vi "Configure_Self_Test.vi"(7 "I2C Channel":u8, 8 "error in":errorcluster, 10 "Self Test":T1 {"Self-Test Control" items=["Self-Test DISABLE"=0, "Self-Test ENABLE"=2]; "Self-Test Sign" items=["Self Test (plus)"=0, "Self Test (minus)"=8]}, 11 "LINX Resource In":T2) -> (0 "error out":errorcluster, 3 "LINX Resource Out":T2)   [LabVIEW 2014, in "LMH-LINX.lvlib" / "LIS331HH.lvlib"]
doc: "This VI is used to configure and enale/disable device self-test\n\n**Author: Stas Legedza"
uses:
  <vilib>/MakerHub/LINX/Public/Sensors/Accelerometer/LIS331HH/LIS331HH.lvlib
  <vilib>/MakerHub/LINX/Private/Type Defs/LINX Ref.ctl
  <vilib>/MakerHub/LINX/Private/Type Defs/Platform.ctl
  <vilib>/MakerHub/LINX/Private/Type Defs/Interface.ctl
  <vilib>/MakerHub/LINX/Private/Device/Type Defs/LINX Device Config.ctl
  <vilib>/MakerHub/LINX/Private/Device/Type Defs/TCP Config.ctl
  <vilib>/MakerHub/LINX/Private/Device/Type Defs/Channels.ctl
  <vilib>/MakerHub/LINX/Private/Local IO/LinxI2cWrite.vi
  <vilib>/MakerHub/LINX/Public/Utilities/Check Channel.vi
  <vilib>/MakerHub/LINX/Private/Utilties/Generate Error.vi
  <vilib>/MakerHub/LINX/LMH-LINX.lvlib
  <vilib>/MakerHub/LINX/Private/Device/Device.lvlib
panel:
  # "OUTPUTS"
  # "INPUTS"
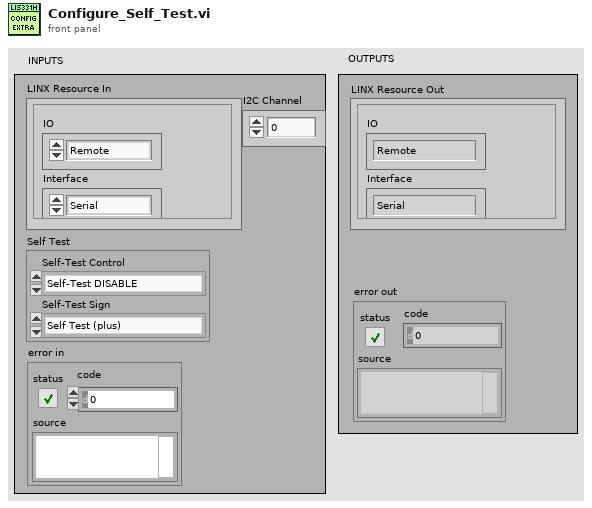
[diagram p1: front panel]
types:
  T1 = cluster{"Self-Test Control":u8, "Self-Test Sign":u8}
  T2 = typedef "LMH-LINX.lvlib/LINX Ref.ctl" = cluster{"IO":T3, "Interface":T4, "LINX Device Config":T5}
  T3 = typedef "LMH-LINX.lvlib/Platform.ctl" = enum16{"Remote", "Local"}
  T4 = typedef "LMH-LINX.lvlib/Interface.ctl" = enum16{"Serial", "TCP"}
  T5 = typedef "LMH-LINX.lvlib/Device.lvlib/LINX Device Config.ctl" = cluster{"Interface":T4, "COM Port":refnum<visa-resource-name>, "TCP Configuration":T6, "Device Family":u8, "Device ID":u8, "Device Name":string, "TCP Ref":refnum<k5>, "Channels":T7}
  T6 = typedef "LMH-LINX.lvlib/Device.lvlib/TCP Config.ctl" = cluster{"IP Address":string, "Port":u16}
  T7 = typedef "LMH-LINX.lvlib/Channels.ctl" = cluster{"DI":u8[], "DO":u8[], "AI":u8[], "AO":u8[], "PWM":u8[], "QE":u8[], "UART":u8[], "I2C 2":u8[], "SPI":u8[], "CAN":u8[], "Servo":u8[], "AI Ref (V)":dbl, "AI Resolution (Bits)":u8, "AO Ref (V)":dbl, "AO Resolution (Bits)":u8}
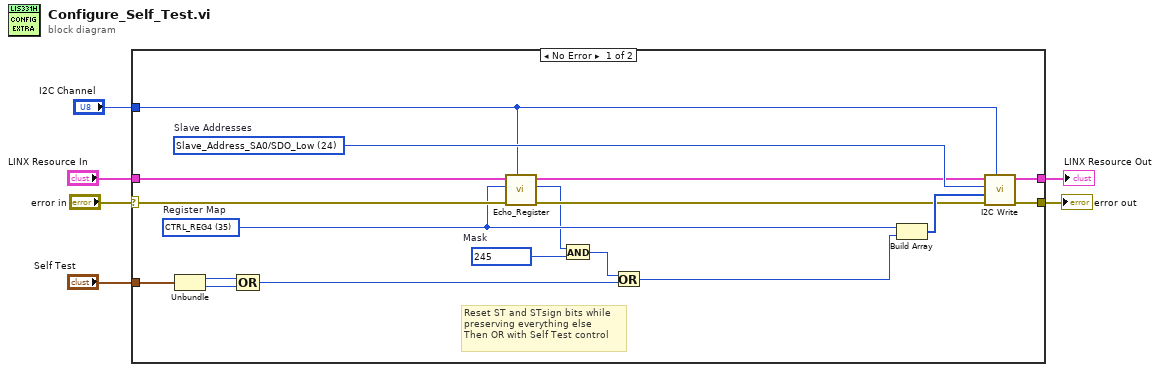
[diagram p0: block diagram]
diagram:
  n1 = case shown="No Error" "error in" {
    selector: "error in" -> [w19 w26]
    tunnel: [w22 w26] -> w5
    tunnel: "LINX Resource In" -> [w20 w25]
    tunnel: "I2C Channel" -> [w16 _]
    tunnel: [w23 w25] -> w2
    tunnel: "Self Test" -> [w10 _]
    frame No Error {
      w13 = u8 245  # Mask
      w21 = u8 24 items=["Slave_Address_SA0/SDO_Low"=24, "Slave_Address_SA0/SDO_High"=25]  # Slave Addresses
      w15 = u8 35 items=["CTRL_REG1"=32, "CTRL_REG2"=33, "CTRL_REG3"=34, "CTRL_REG4"=35, "CTRL_REG5"=36, "HP_FILTER_RESET"=37, "REFERENCE"=38, "STATUS_REG"=39, "OUT_X_L"=40, "OUT_X_H"=41, "OUT_Y_L"=42, "OUT_Y_H"=43, "OUT_Z_L"=44, "OUT_Z_H"=45, "INT1_CFG"=48, "INT1_SOURCE"=49, "INT1_THS"=50, "INT1_DURATION"=51, "INT2_CFG"=52, "INT2_SOURCE"=53, "INT2_THS"=54, "INT2_DURATION"=55]  # Register Map
      # "Reset ST and STsign bits while \npreserving everything else\nThen OR with Self Test control"
      n2 = Unbundle(w10) -> ("Self-Test Control"=w9:u8, "Self-Test Sign"=w8:u8)
      n3 = Compound Arithmetic op=OR(w9, w8) -> (w7:u8)
      n4 = call <vilib>:"Echo_Register.vi"("I2C Channel"=w16, "error in (no error)"=w19, "Register to Echo"=w15, "LINX Resource In"=w20) -> ("error out"=w17:errorcluster, "Register Word"=w14:u8, "LINX Resource Out"=w18:T2)  [unwired: 5 in]
      n5 = And(x=w14, y=w13) -> (x .and. y?=w12:u8)
      n6 = Or(x=w12, y=w7) -> (x .or. y?=w11:u8)
      n7 = Build Array(w15, w11) -> (w24:u8[])
      n8 = call <vilib>:"I2C Write.vi"("I2C Channel"=w16, "Error In"=w17, "Data"=w24, "I2C Slave Address (0)"=w21, "LINX Resource"=w18) -> ("Error Out"=w22:errorcluster, "LINX Resource"=w23:T2)  [unwired: 5 in]
    }
    frame Error {
    }
  }
  "error out" <- w5
  "LINX Resource Out" <- w2
